vi "Demo_2.vi"() -> ()   [LabVIEW 2017]
uses:
  Components/ViPER.lvlibp/ViPER.lvclass
panel:
  out "error out":errorcluster
  in  "Config XML":string="<?xml version=\"1.0\" encoding=\"UTF-8\" standalone=\"no\" ?>\n<Object>\n\n  <Name>panel</Name>\n\n  <Class>DUT_Handler_Simple</Class>\n\n</Object>\n"
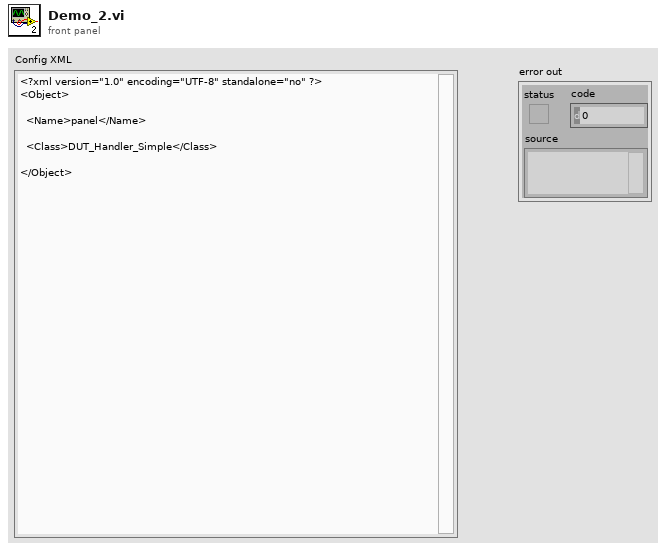
[diagram p1: front panel]
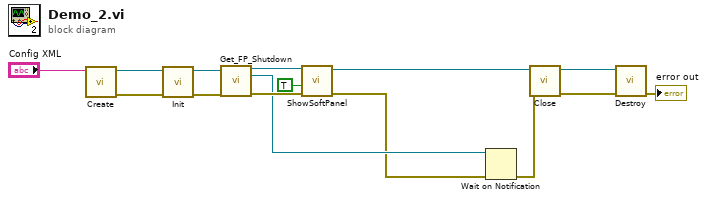
[diagram p0: block diagram]
diagram:
  n1 = call "Create.vi"("Config XML"="Config XML") -> ("error out"=w15:errorcluster, "reference out"=w14:refnum<class "ViPER.lvclass">)  [unwired: 9 in]
  n2 = call-dynamic "Init.vi"("error in (no error)"=w15, "reference in"=w14) -> ("error out"=w12:errorcluster, "reference out"=w11:refnum<class "ViPER.lvclass">)  [unwired: 8 in]
  n3 = call "Get_FP_Shutdown.vi"("ViKing_Base in"=w11, "error in (no error)"=w12) -> ("ViKing_Base out"=w9:refnum<class "ViPER.lvclass">, "SoftFP_Shutdown"=w5:refnum<notifier>, "error out"=w10:errorcluster)  [unwired: 9 in, 2 out]
  n4 = call-dynamic "ShowSoftPanel.vi"("error in (no error)"=w10, "Floating"=TRUE, "Driver in"=w9) -> ("error out"=w1:errorcluster, "Driver out"=w3:refnum<class "ViPER.lvclass">)  [unwired: 6 in, 1 out]
  n5 = Wait on Notification(notifier=w5, error in (no error)=w1) -> (error out=w4:errorcluster)  [unwired: 2 in, 3 out]
  n6 = call-dynamic "Close.vi"("error in (no error)"=w4, "reference in"=w3) -> ("error out"=w8:errorcluster, "reference out"=w7:refnum<class "ViPER.lvclass">)  [unwired: 8 in]
  n7 = call "Destroy.vi"("error in (no error)"=w8, "reference in"=w7) -> ("error out"=→"error out":errorcluster)  [unwired: 9 in]
